vi "I2C Burst Write.vi"(8 "error in (no error)":errorcluster, 9 "data":string, 10 "nBytes":i32, 11 "i2cAddress":u8) -> (0 "error out":errorcluster, 1 "data out":string, 3 "function return":u32)   [LabVIEW 2014, in "atmcd32d.lvlib"]
doc: "unsigned int WINAPI I2CBurstWrite(BYTE i2cAddress, long nBytes, BYTE * data);"
uses:
  atmcd32d.lvlib
  atmcd32d.dll
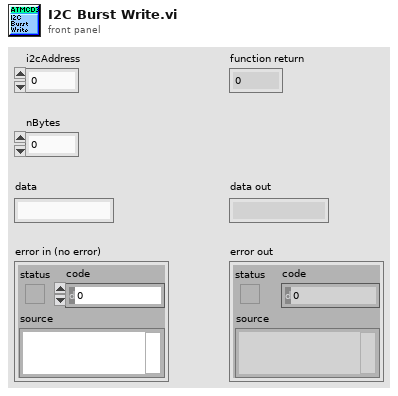
[diagram p1: front panel]
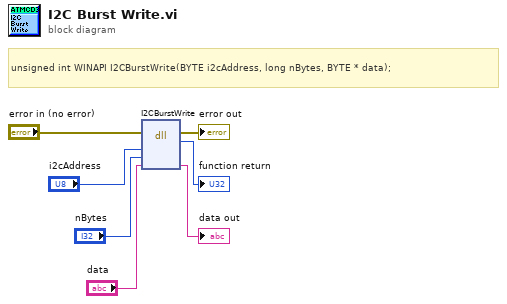
[diagram p0: block diagram]
diagram:
  # "unsigned int WINAPI I2CBurstWrite(BYTE i2cAddress, long nBytes, BYTE * data);"
  n1 = dll-call lib="C:/Users/Bakir/Documents/Lambda2-Testing/lib/Andorlib/atmcd32d.*" fn="I2CBurstWrite"(error in="error in (no error)", "i2cAddress"="i2cAddress", "nBytes"="nBytes", "data"="data") -> (error out=→"error out":errorcluster, →"function return":u32, "data"=→"data out":string)  [unwired: 4 in, 1 out]
